vi "DrawPlayfield_Clear.vi"(2 "Player":u8) -> ()   [LabVIEW 2018]
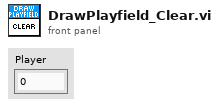
[diagram p1: front panel]
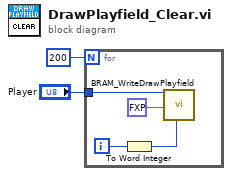
[diagram p0: block diagram]
diagram:
  n1 = for {
    N: 200 -> [_]
    tunnel: "Player" -> [w6]
    i -> [w4]
    n2 = To Word Integer(number=w4) -> (16bit integer=w3:i16)
    n3 = call "BRAM_WriteDrawPlayfield.vi"("Player IN"=w6, "Data"=fxp<+,3,3> 0.0, "Address"=w3) -> ()  [unwired: 16 in, 1 out]
  }
